vi "ConstructStackTest.vi"() -> ()   [LabVIEW 2009]
uses:
  <vilib>/rvi/interface/nirviOpenFPGA/nirviOpenFPGA.xnode
  FPGA_Control/FPGA Bitfiles/AOD Control.lvproj_FPGA Target_AOD Control (FPGA)~D2.lvbitx
  FPGA_Control/AOD Control (FPGA).vi
  <vilib>/rvi/interface/RandomDataEmulation/nirviRandomDataOpen.vi
  <vilib>/rvi/interface/nirviOpenFPGA/nirviOpenFPGA.ctl
  <vilib>/rvi/interface/nirviOpenFPGA/nirviopenstate.ctl
  <vilib>/picture/picture.llb/imagedata.ctl
  <vilib>/rvi/interface/common/nirviIntfCommonState.ctl
  <vilib>/rvi/interface/common/nirviIntfModes.ctl
  C:/Program Files/National Instruments/LabVIEW 2009/resource/RVI/emulation/niLvFpgaEmulationMode.ctl
  <vilib>/eio/XNode/Errors/EIOXNodeErrorStruct.ctl
  <vilib>/eio/XNode/Errors/EIOXNodeInternalErrorTypes.ctl
  <vilib>/eio/XNode/Errors/EIOXNodeUserErrorTypes.ctl
  <vilib>/XNodeSupport/XNodeRect32.ctl
  <vilib>/XNodeSupport/XNodeInt.ctl
  <vilib>/XNodeSupport/XNodeTerms.ctl
  <vilib>/XNodeSupport/XNodeTerm.ctl
  <vilib>/XNodeSupport/XNodeString.ctl
  <vilib>/XNodeSupport/XNodeVariant.ctl
  <vilib>/XNodeSupport/XNodeBool.ctl
  <vilib>/rvi/interface/nirviReadWriteControl/nirviReadWriteControl.xnode
  <vilib>/rvi/interface/nirviMethod/nirviMethod.xnode
  <vilib>/rvi/interface/RandomDataEmulation/nirviRandomDataDMAMethods.vi
  <vilib>/rvi/interface/common/niFpgaNodeNameForErrorReporting.ctl
  <vilib>/userdefined/High Color/nirio_resource_hc.ctl
  <vilib>/XNodeSupport/NI_XNodeSupport.lvlib
panel:
  in  "ReadSize":i32
  out "Array":T1[][](array[plugin-control])
  in  "stop":bool
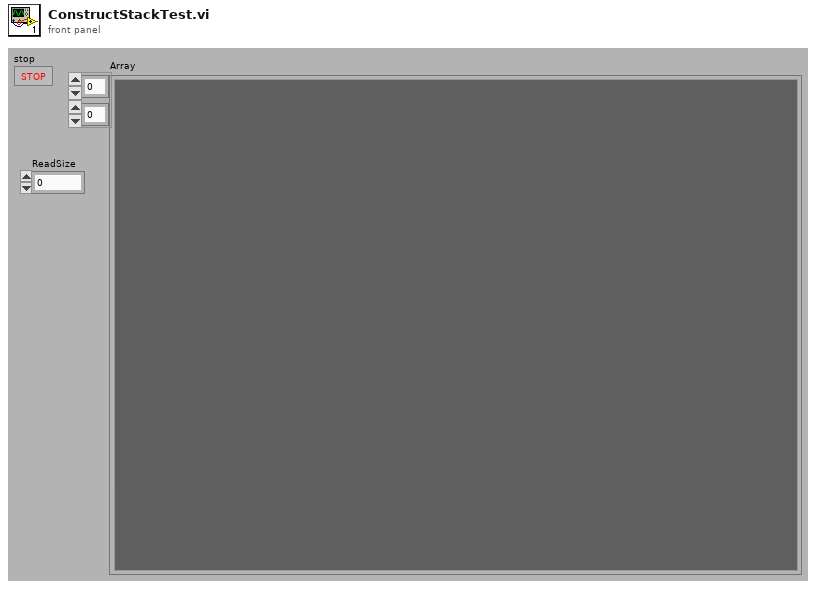
[diagram p1: front panel]
types:
  T1 = typedef "IMAQ Image.ctl" = refnum<image>
  T2 = typedef "Image Type" = u32
  T3 = typedef "niFpgaNodeNameForErrorReporting.ctl" = enum16{"Open FPGA VI Reference", "Read/Write Control", "Invoke Method: Abort", "Invoke Method: Acknowledge IRQ", "Invoke Method: Download", "Invoke Method: FIFO.Configure", "Invoke Method: FIFO.Read", "Invoke Method: FIFO.Start", "Invoke Method: FIFO.Stop", "Invoke Method: FIFO.Write", "Invoke Method: Reset", "Invoke Method: Run", "Invoke Method: Wait on IRQ", "Close FPGA VI Reference"}
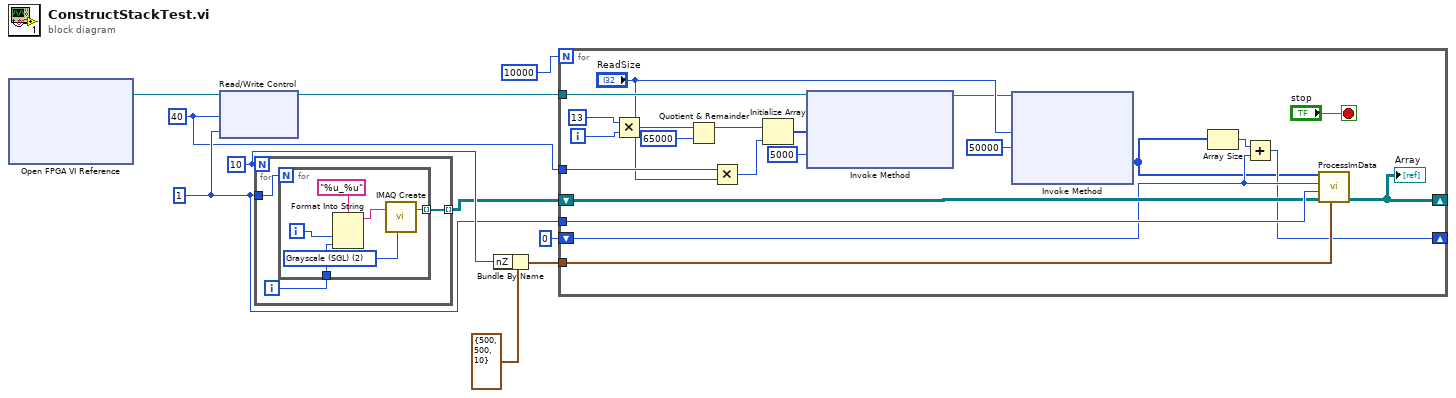
[diagram p0: block diagram]
diagram:
  w1 = u32 40 ("Downsample")
  w10 = 10
  w2 = u32 1 ("NumChans")
  n1 = xnode "Open FPGA VI Reference"() -> ("FPGA VI Reference Out"=w4:refnum<k20>)  [unwired: 2 in, 1 out]
  n2 = xnode "Read/Write Control"("FPGA VI Reference In"=w4, "Downsample"=w1, "Channels"=w2) -> ("FPGA VI Reference Out"=w3:refnum<k20>)  [unwired: 1 in, 1 out]
  n3 = for {
    N: w10 -> [_]
    tunnel: [w13] -> w7 mode=indexing
    tunnel: w2 -> [w12]
    i -> [w11]
    n4 = for {
      N: w12 -> [_]
      tunnel: [w19] -> w13 mode=indexing
      tunnel: w11 -> [w16]
      i -> [w17]
      w14 = T2 2 items=["Grayscale (U8)", "Grayscale (I16)", "Grayscale (SGL)", "Complex (CSG)", "RGB (U32)", "HSL (U32)", "RGB (U64)", "Grayscale (U16)"] ("Image Type")
      n5 = Format Into String(format string="%u_%u", w17, w16) -> (resulting string=w15:string)  [unwired: 2 in, 1 out]
      n6 = call "IMAQ Create"("Image Name"=w15, "Image Type"=w14) -> ("New Image"=w19:T1)  [unwired: 3 in, 1 out]
    }
  }
  n7 = Bundle By Name(cluster=cluster{"nX":u32, "nY":u32, "nZ":u32} {"nX"=500, "nY"=500, "nZ"=10} ("StackSize"), "nZ"=w10) -> (w8:cluster{"nX":u32, "nY":u32, "nZ":u32})
  n8 = for {
    N: 10000 -> [_]
    tunnel: w2 -> [w41]
    tunnel: w8 -> [w40]
    shift-right: [w35] -> _
    shift-left: 0 -> [w37]
    shift-right: [w34] -> _
    shift-left: w7 -> [w39]
    tunnel: w3 -> [w28]
    tunnel: w1 -> [w26]
    i -> [w33]
    stop <- "stop" stop-if-true
    n9 = Multiply(x=13, y=w33) -> (x*y=w31:i32)
    n10 = Quotient & Remainder(x=w31, y=65000) -> (x-y*floor(x/y)=w29:i32)  [unwired: 1 out]
    n11 = Multiply(x=w26, y="ReadSize") -> (x*y=w25:u32)
    n12 = Initialize Array(w29, w25) -> (w27:i32[])
    n13 = xnode "Invoke Method"("FPGA VI Reference In"=w28, "Data"=w27, "Timeout (ms)"=5000) -> ("FPGA VI Reference Out"=w23:refnum<k20>)  [unwired: 1 in, 2 out]
    n14 = xnode "Invoke Method"("FPGA VI Reference In"=w23, "Number of Elements"="ReadSize", "Timeout (ms)"=50000) -> ("Data"=w22:i32[])  [unwired: 1 in, 3 out]
    n15 = Array Size(array=w22) -> (size(s)=w36:i32)
    n16 = Add(x=w36, y=w37) -> (x+y=w35:i32)
    n17 = call "ProcessImData.vi"("StackSize"=w40, "Image Array In"=w39, "NumChans"=w41, "StartingNum"=w37, "Data"=w22) -> ("Image Array Out"=w34:T1[][])  [unwired: 5 in, 1 out]
    "Array" <- w34
  }
